vi "update_progress_bar.vi"(8 "error in (no error)":errorcluster, 10 "progress ref":refnum<vi>, 11 "Volumes in":refnum<class "Volumes.lvclass">) -> (0 "error out":errorcluster, 3 "Volumes out":refnum<class "Volumes.lvclass">)   [LabVIEW 2024, in "CLZ_to_ComicVine.lvlib" / "Volumes.lvclass"]
uses:
  Volumes.lvclass
  Volumes.lvclass/Volumes.ctl
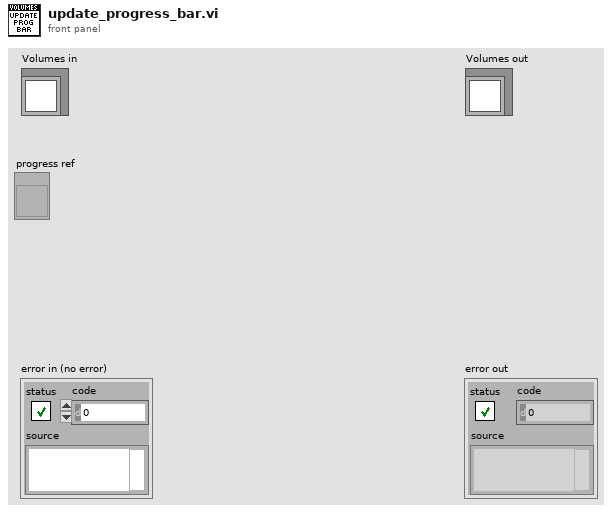
[diagram p1: front panel]
types:
  T1 = typedef "CLZ_to_ComicVine.lvlib/Volumes.lvclass/volume--cluster.ctl" = cluster{"id":i32, "name":string, "issue set":set{string}, "matched":bool}
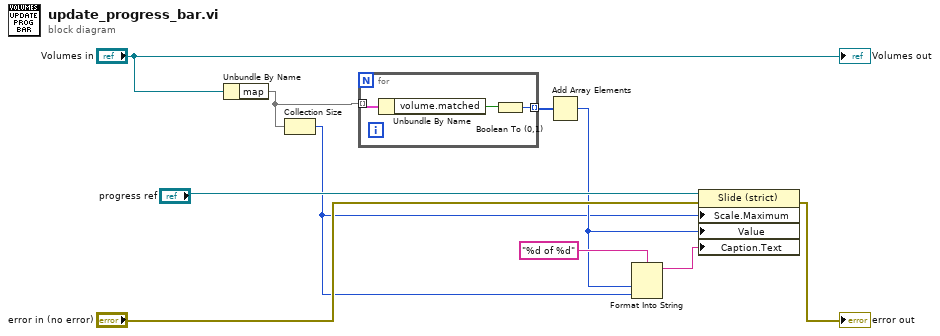
[diagram p0: block diagram]
diagram:
  n1 = Unbundle By Name("Volumes in") -> ("map"=w7:map{i32, T1})
  n2 = Collection Size(1:w7) -> (0:w3:i32)
  n3 = for {
    tunnel: w7 -> [w13] mode=indexing
    tunnel: [w11] -> w6 mode=indexing
    n4 = Unbundle By Name(w13) -> ("volume.matched"=w12:bool)
    n5 = Boolean To (0,1)(Boolean=w12) -> (0, 1=w11:i16)
  }
  n6 = Add Array Elements(numeric array=w6) -> (sum=w4:i16)
  n7 = Format Into String(format string="%d of %d", w4, w3) -> (resulting string=w1:string)  [unwired: 2 in, 1 out]
  n8 = property class="Slide (strict)"(reference="progress ref", error in="error in (no error)", "Scale.Maximum"=w3, "Value"=w4, "Caption.Text"=w1) -> (error out=→"error out":errorcluster)  [unwired: 1 out]
  "Volumes out" <- "Volumes in"
